vi "Scale Waveform Amplitude between -1 and 1.vi"(7 "AmpGain":i32=1, 9 "Offset":dbl, 10 "Gain":dbl, 11 "Waveform Amplitude In (V)":dbl) -> (0 "error out":errorcluster, 3 "Waveform Amplitude Out (-1 to 1)":dbl)   [LabVIEW 2013]
doc: "This VI Converts the amplitude of a requested waveform to the range of -1 to 1 to be accepted by AWG's waveform creator VIs based on the Gain and Offset of the AWG"
uses:
  <vilib>/Utility/error.llb/Error Cluster From Error Code.vi
  <vilib>/ErrorRing/Error Ring.xnode
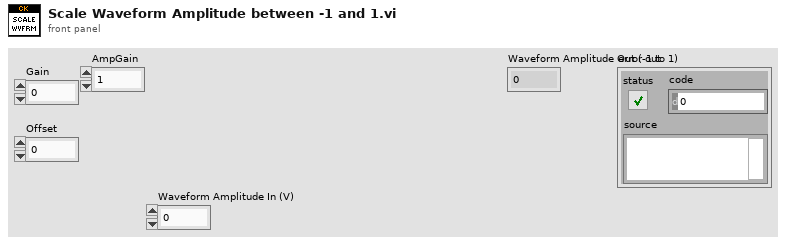
[diagram p1: front panel]
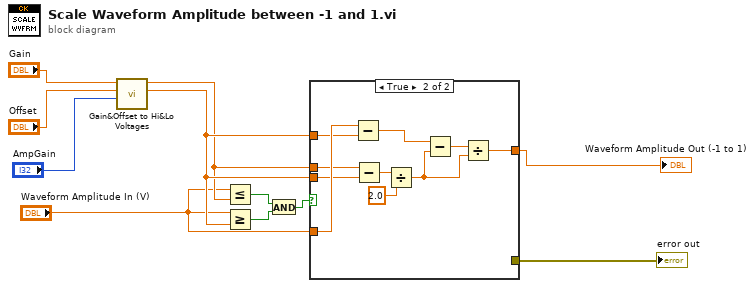
[diagram p0: block diagram]
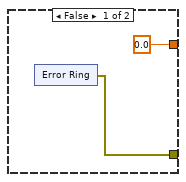
[diagram p2: hidden frame]
diagram:
  n1 = call "Gain&Offset to Hi&Lo Voltages.vi"("AmpGain"="AmpGain", "AWG Offset"="Offset", "AWG Gain"="Gain") -> ("VLo"=w5:dbl, "VHi"=w4:dbl)  [unwired: 7 in]
  n2 = Less Or Equal?(x="Waveform Amplitude In (V)", y=w4) -> (x <= y?=w3:bool)
  n3 = Greater Or Equal?(x="Waveform Amplitude In (V)", y=w5) -> (x >= y?=w2:bool)
  n4 = And(x=w3, y=w2) -> (x .and. y?=w6:bool)
  n5 = case shown="True" w6 {
    tunnel: "Waveform Amplitude In (V)" -> [_ w28]
    tunnel: w5 -> [_ w27]
    tunnel: w4 -> [_ w26]
    tunnel: w5 -> [_ w25]
    tunnel: [0.0 w24] -> w8
    tunnel: [w12 _] -> w7
    frame False {
      n6 = xnode "Error Ring"() -> ("error out"=w12:errorcluster)
    }
    frame True {
      n7 = Subtract(x=w28, y=w27) -> (x-y=w21:dbl)
      n8 = Subtract(x=w26, y=w25) -> (x-y=w23:dbl)
      n9 = Divide(x=w23, y=2.0) -> (x/y=w20:dbl)
      n10 = Subtract(x=w21, y=w20) -> (x-y=w19:dbl)
      n11 = Divide(x=w19, y=w20) -> (x/y=w24:dbl)
    }
  }
  "error out" <- w7
  "Waveform Amplitude Out (-1 to 1)" <- w8
